vi "3 Mirror Engine.vi"(0 "Unique Notifier Name":string, 11 "DAQmx AO Lines":string[](array[string])) -> ()   [LabVIEW 2020]
uses:
  3 Mirror Scan Type Defs/3 Mirror Scan Note Type.ctl
  3 Mirror Scan Type Defs/3 Mirror Scan Actions.ctl
  3 Mirror Scan Type Defs/3 Mirror Scan Cal Data.ctl
  <vilib>/DAQmx/write.llb/DAQmx Write (Analog 1D Wfm NChan NSamp).vi
  <vilib>/DAQmx/write.llb/DAQmx Write (Analog 1D DBL NChan 1Samp).vi
  <vilib>/DAQmx/create/channels.llb/DAQmx Create Channel (AO-Voltage-Basic).vi
  <vilib>/DAQmx/configure/timing.llb/DAQmx Timing (Sample Clock).vi
  <vilib>/DAQmx/miscellaneous.llb/DAQmx Fill In Error Info.vi
  <resource>/objmgr/daqmx.rc
panel:
  out "Last Error":errorcluster
  in  "Quit":bool
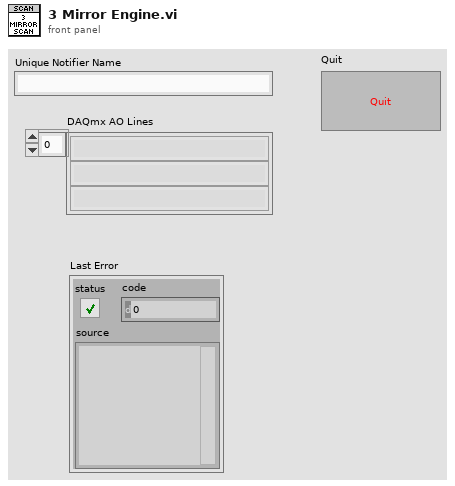
[diagram p1: front panel]
types:
  T1 = typedef "3 Mirror Scan Cal Data.ctl" = cluster{"XCenter":dbl, "YCenter":dbl, "M1_Px_Per_Volt":dbl, "M2_Px_Per_Volt":dbl, "MirrorCoupling":dbl, "Phase01":dbl, "Phase02":dbl, "Phase03":dbl}
  T2 = typedef "3 Mirror Scan Actions.ctl" = enum16{"Idle", "Scan Timed", "Scan Live", "Convert ROI", "Run Scan", "Exit Loop", "Quit"}
  T3 = typedef "3 Mirror Scan Note Type.ctl" = cluster{"Actions":T2, "Global Rectangle":i32[], "Running":bool, "Scan Frequency (Hz)":dbl, "Scan Time (s)":dbl}
  T4 = typedef "3 Mirror Scan ROI Voltage Data.ctl" = cluster{"X Freq (Hz)":dbl, "Y Freq (Hz)":dbl, "X Offset (V)":dbl, "X Amp (V)":dbl, "Y Offset (V)":dbl, "Y Amp (V)":dbl}
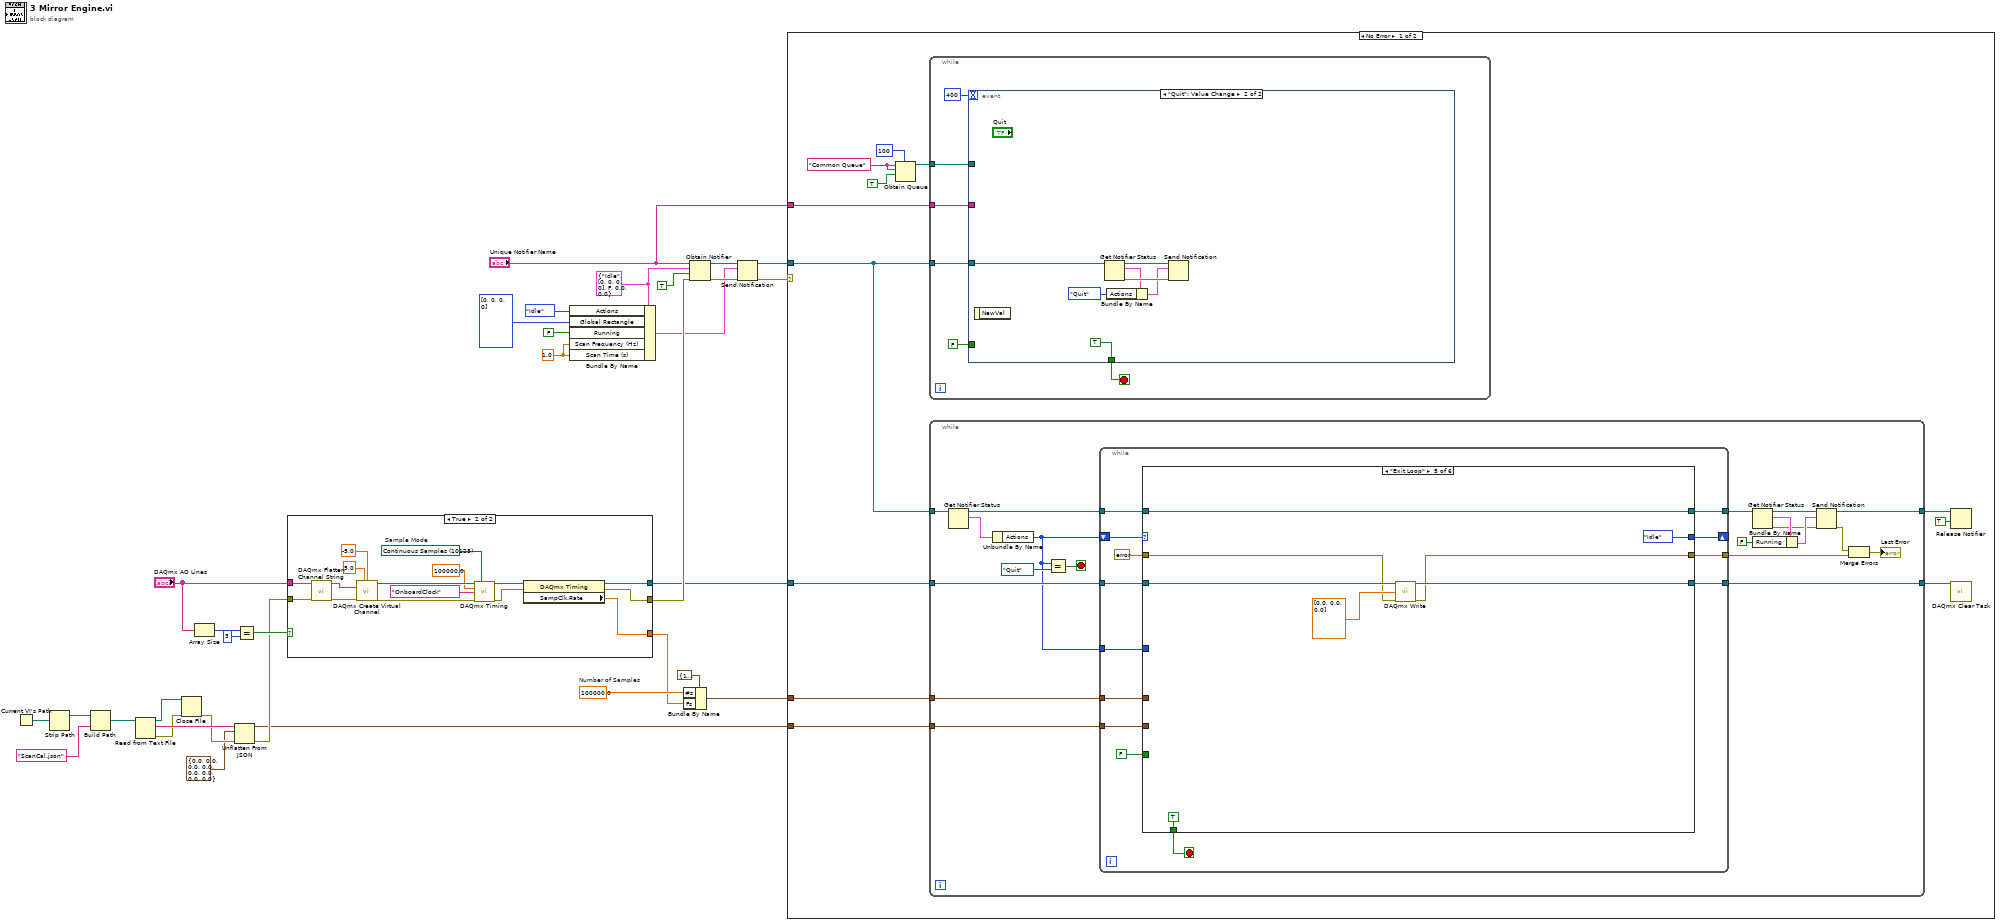
[diagram p0: block diagram]
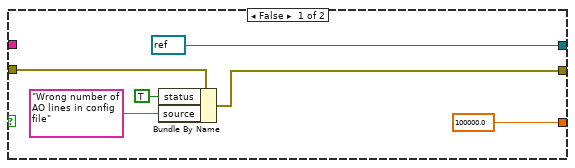
[diagram p2: hidden frame]
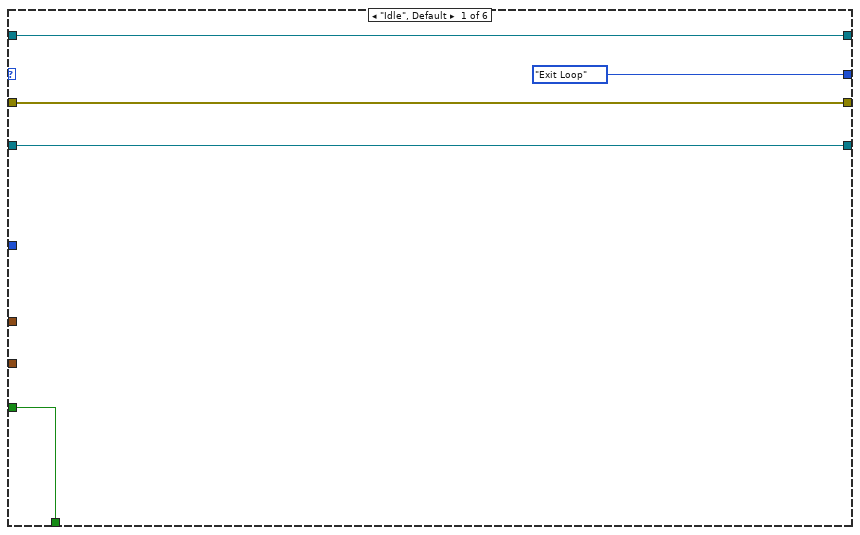
[diagram p3: hidden frame]
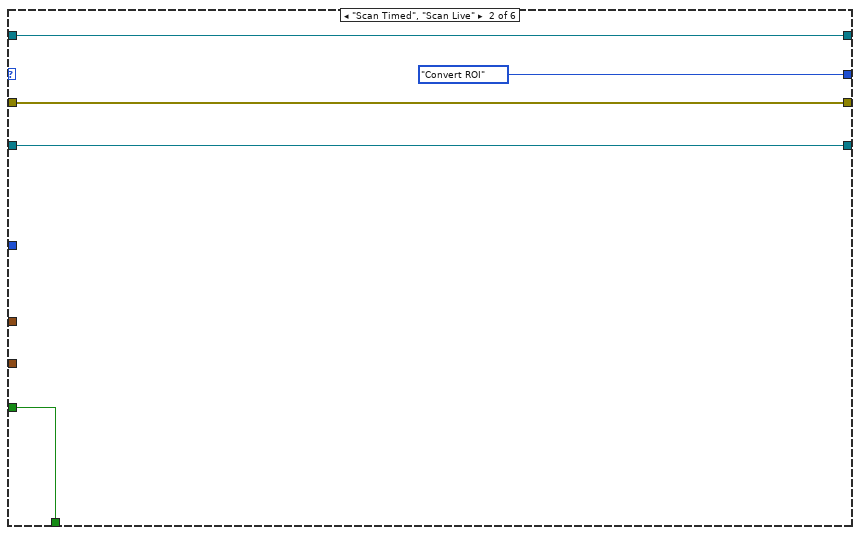
[diagram p4: hidden frame]
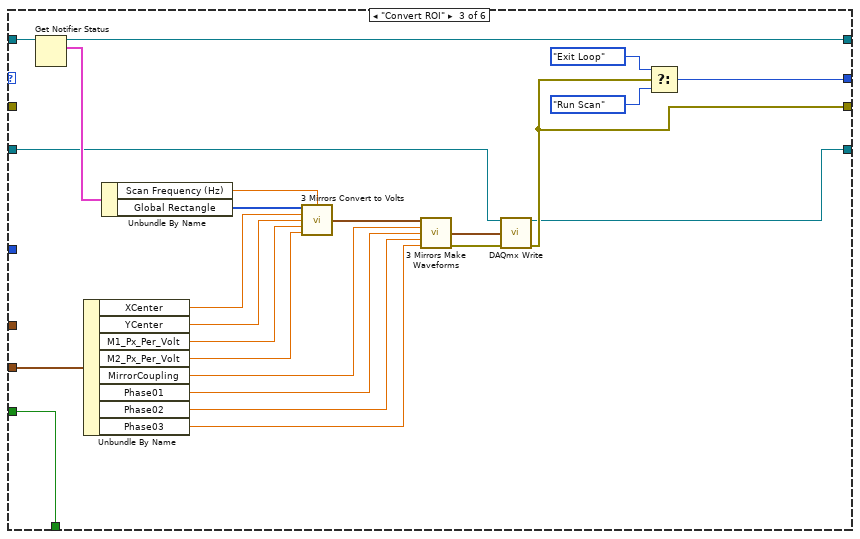
[diagram p5: hidden frame]
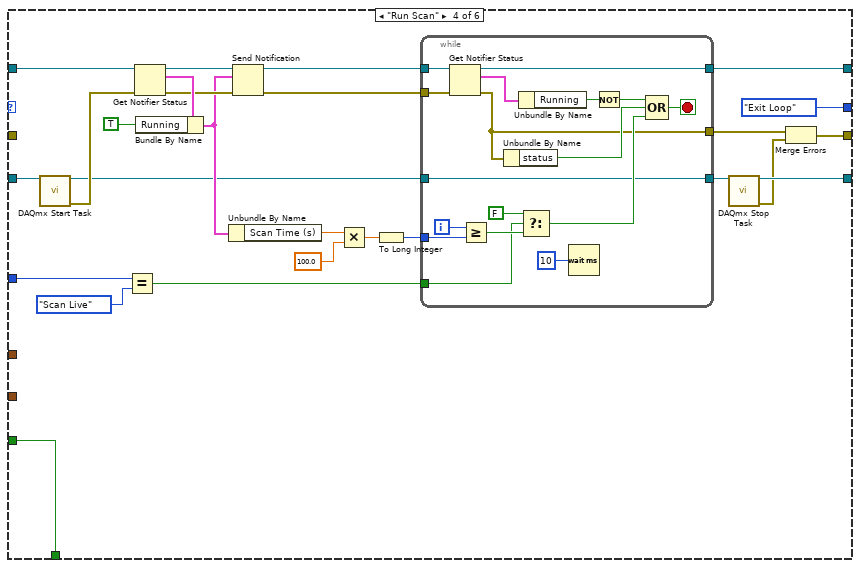
[diagram p6: hidden frame]
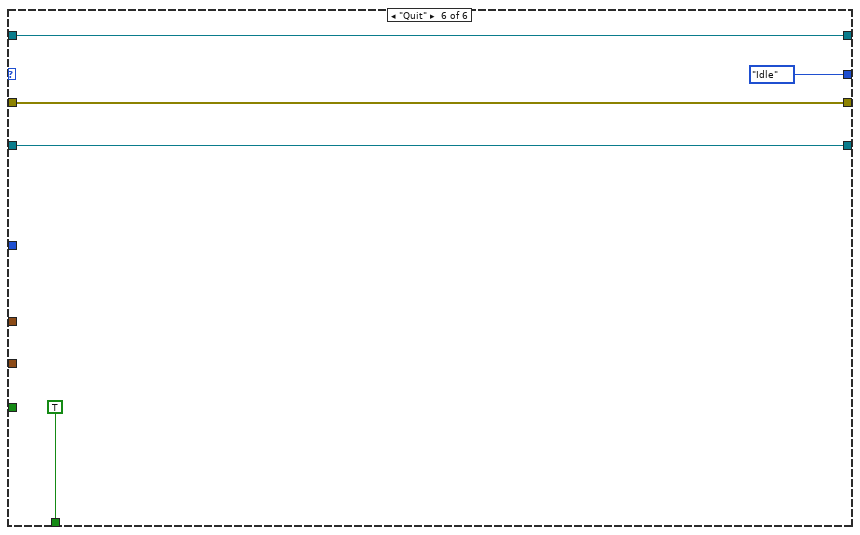
[diagram p7: hidden frame]
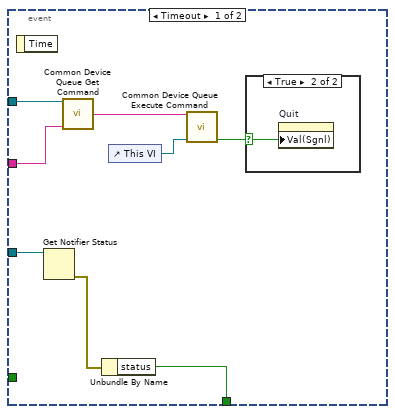
[diagram p8: hidden frame]
diagram:
  w15 = 1.0 ("Scan Frequency (Hz)")
  w19 = T3 {"Actions"=enum."Idle", "Global Rectangle"=[0, 0, 0, 0], "Running"=FALSE, "Scan Frequency (Hz)"=0.0, "Scan Time (s)"=0.0} ("3 Mirror Notifier")
  w21 = 100000.0  # Number of Samples
  n1 = Current VI's Path() -> (path=w12:path)
  n2 = Strip Path(path=w12) -> (stripped path=w11:path)  [unwired: 1 out]
  n3 = Build Path(base path=w11, name or relative path="ScanCal.json") -> (appended path=w9:path)
  n4 = Read from Text File(file (use dialog)=w9) -> (refnum out=w7:refnum<file>, text=w8:string, error out=w6:errorcluster)  [unwired: 3 in, 1 out]
  n5 = Close File(refnum=w7, error in=w6) -> (error out=w5:errorcluster)  [unwired: 1 out]
  n6 = Array Size(array="DAQmx AO Lines") -> (size(s)=w27:i32)
  n7 = Unflatten From JSON(JSON string=w8, type and defaults=T1 {"XCenter"=0.0, "YCenter"=0.0, "M1_Px_Per_Volt"=0.0, "M2_Px_Per_Volt"=0.0, "MirrorCoupling"=0.0, "Phase01"=0.0, "Phase02"=0.0, "Phase03"=0.0} ("ScanCalibration"), error in (no error)=w5) -> (value=w2:T1, error out=w3:errorcluster)  [unwired: 4 in]
  n8 = Equal?(x=w27, y=3) -> (x = y?=w25:bool)
  n9 = case shown="True" w25 {
    tunnel: "DAQmx AO Lines" -> [_ w55]
    tunnel: w3 -> [w39 w54]
    tunnel: [w35 w41] -> w23
    tunnel: [refnum<k21> refnum ("task out") w42] -> w13
    tunnel: [100000.0 ("Sample Rate") w40] -> w20
    frame False {
      n10 = Bundle By Name(cluster=w39, "status"=TRUE, "source"="Wrong number of AO lines in config file") -> (w35:errorcluster)
    }
    frame True {
      w51 = 10123 items=["Finite Samples"=10178, "Continuous Samples"=10123, "Hardware Timed Single Point"=12522]  # Sample Mode
      n11 = call <vilib>:"DAQmx Flatten Channel String.vi"("names in"=w55, "error in"=w54) -> ("names out"=w46:string, "error out"=w45:errorcluster)  [unwired: 12 in]
      n12 = call-poly <vilib>:"DAQmx Create Virtual Channel.vi"("maximum value"=5.0 ("Max Voltage"), "minimum value"=-5.0 ("Min Voltage"), "physical channels"=w46, "error in"=w45) -> ("task out"=w53:refnum<k21>, "error out"=w52:errorcluster)  [unwired: 10 in]
      n13 = call-poly <vilib>:"DAQmx Timing.vi"("task/channels in"=w53, "sample mode"=w51, "rate"=100000.0 ("Sample Rate"), "source"=tag "OnboardClock" ("Sample Clock Source"), "error in"=w52) -> ("task out"=w44:refnum<k21>, "error out"=w43:errorcluster)  [unwired: 9 in]
      n14 = property class="DAQmx Timing"(reference=w44, error in=w43) -> (reference out=w42:refnum<k21>, error out=w41:errorcluster, "SampClk.Rate"=w40:dbl)
    }
  }
  n15 = Bundle By Name(cluster=w19, "Actions"=3_Mirror_Scan_Actions."Idle", "Global Rectangle"=i32[] [0, 0, 0, 0], "Running"=FALSE, "Scan Frequency (Hz)"=w15, "Scan Time (s)"=w15) -> (w14:T3)
  n16 = Bundle By Name(cluster=cluster{"Fs":dbl, "#s":dbl} {"Fs"=1000.0, "#s"=1000.0} ("sampling info"), "#s"=w21, "Fs"=w20) -> (w1:cluster{"Fs":dbl, "#s":dbl})
  n17 = Obtain Notifier(name (unnamed)="Unique Notifier Name", notification data type=w19, create if not found? (T)=TRUE, error in (no error)=w23) -> (notifier out=w32:refnum<notifier>, error out=w31:errorcluster)  [unwired: 1 out]
  n18 = Send Notification(notification=w14, notifier=w32, error in (no error)=w31) -> (notifier out=w29:refnum<notifier>, error out=w30:errorcluster)
  n19 = case shown="No Error" w30 {
    tunnel: w29 -> [w62 _]
    tunnel: "Unique Notifier Name" -> [w63 _]
    tunnel: w13 -> [w61 _]
    tunnel: w2 -> [w58 _]
    tunnel: w1 -> [w57 _]
    frame No Error {
      w67 = "Common Queue" ("Unique Notifier Name")
      n20 = Obtain Queue(max queue size (-1, unlimited)=100, name (unnamed)=w67, element data type=w67, create if not found? (T)=TRUE) -> (queue out=w64:refnum<queue>)  [unwired: 1 in, 2 out]
      n21 = while {
        tunnel: w62 -> [w196]
        tunnel: w64 -> [w193]
        tunnel: w63 -> [w192]
        stop <- w194 stop-if-true
        n22 = event shown="[1] \"Quit\": Value Change" {
          selector: _ -> [_ _]
          dyn-events: _ -> [_ _]
          timeout: 400 -> [_ _]
          tunnel: w196 -> [w204 w207]
          tunnel: [w202 TRUE ("status")] -> w194
          tunnel: w193 -> [w198 _]
          tunnel: w192 -> [w197 _]
          tunnel: FALSE ("status") -> [_ _]
          event Timeout {
            n23 = event-data() -> ()  [unwired: 1 in, 1 out]
            n24 = Get Notifier Status(notifier=w204) -> (error out=w203:errorcluster)  [unwired: 1 in, 4 out]
            n25 = call "Common Device Queue Get Command.vi"("Common Queue"=w198, "Notifier Name"=w197) -> ("Command"=w200:string)  [unwired: 12 in, 1 out]
            n26 = Unbundle By Name(w203) -> ("status"=w202:bool)
            n27 = control-ref of="This VI"() -> (w199:refnum<vi>)
            n28 = call "Common Device Queue Execute Command.vi"("Common Command"=w200, "VI Refnum"=w199) -> ("Quit?"=w201:bool)  [unwired: 12 in, 1 out]
            n29 = case shown="True" w201 {
              selector: w201 -> [_ w205]
              frame False {
              }
              frame True {
                n30 = property on="Quit" class="Bool (strict)"("Val(Sgnl)"=w205) -> ()  [unwired: 2 in, 2 out]
              }
            }
          }
          event "Quit": Value Change {
            n31 = event-data() -> ()  [unwired: 1 in, 1 out]
            n32 = Get Notifier Status(notifier=w207) -> (notifier out=w208:refnum<notifier>, current notification=w209:T3, error out=w211:errorcluster)  [unwired: 1 in, 2 out]
            n33 = Bundle By Name(cluster=w209, "Actions"=3_Mirror_Scan_Actions."Quit") -> (w210:T3)
            n34 = Send Notification(notification=w210, notifier=w208, error in (no error)=w211) -> ()  [unwired: 2 out]
          }
        }
      }
      n35 = while {
        tunnel: w62 -> [w87]
        tunnel: w61 -> [w82]
        tunnel: [w75] -> w59
        tunnel: w58 -> [w73]
        tunnel: w57 -> [w74]
        tunnel: [w71] -> w56
        stop <- w84 stop-if-true
        n36 = Get Notifier Status(notifier=w87) -> (notifier out=w83:refnum<notifier>, current notification=w86:T3)  [unwired: 1 in, 3 out]
        n37 = Unbundle By Name(w86) -> ("Actions"=w72:T2)
        n38 = Equal?(x=w72, y=3_Mirror_Scan_Actions."Quit") -> (x = y?=w84:bool)
        n39 = while {
          shift-right: [w95] -> _
          shift-left: w72 -> [w99]
          tunnel: w83 -> [w97]
          tunnel: w82 -> [w96]
          tunnel: [w94] -> w81
          tunnel: w74 -> [w93]
          tunnel: w73 -> [w92]
          tunnel: w72 -> [w91]
          tunnel: [w90] -> w71
          tunnel: [w89] -> w70
          stop <- w98 stop-if-true
          n40 = case shown="\"Exit Loop\"" w99 {
            tunnel: FALSE -> [w105 w110 w134 w160 _ _]
            tunnel: [w105 w110 w134 w160 TRUE TRUE] -> w98
            tunnel: w97 -> [w103 w108 w133 w154 w179 w188]
            tunnel: w96 -> [w101 w106 w118 w159 w184 w187]
            tunnel: [3_Mirror_Scan_Actions."Exit Loop" ("y") 3_Mirror_Scan_Actions."Convert ROI" ("y") w114 3_Mirror_Scan_Actions."Exit Loop" ("y") 3_Mirror_Scan_Actions."Idle" ("y") 3_Mirror_Scan_Actions."Idle" ("y")] -> w95
            tunnel: [w103 w108 w131 w139 w179 w188] -> w94
            tunnel: w93 -> [_ _ _ _ _ _]
            tunnel: w92 -> [_ _ w130 _ _ _]
            tunnel: w91 -> [_ _ _ w152 _ _]
            tunnel: [w101 w106 w111 w140 w182 w187] -> w90
            tunnel: [w102 w107 w112 w135 w180 w186] -> w89
            tunnel: errorcluster {"status"=FALSE, "code"=0, "source"=""} ("error IO") -> [w102 w107 _ _ w181 w186]
            frame "Idle", Default {
            }
            frame "Scan Timed", "Scan Live" {
            }
            frame "Convert ROI" {
              n41 = Get Notifier Status(notifier=w133) -> (notifier out=w131:refnum<notifier>, current notification=w132:T3)  [unwired: 1 in, 3 out]
              n42 = Unbundle By Name(w130) -> ("XCenter"=w124:dbl, "YCenter"=w127:dbl, "M1_Px_Per_Volt"=w126:dbl, "M2_Px_Per_Volt"=w125:dbl, "MirrorCoupling"=w122:dbl, "Phase01"=w121:dbl, "Phase02"=w120:dbl, "Phase03"=w119:dbl)
              n43 = Unbundle By Name(w132) -> ("Scan Frequency (Hz)"=w128:dbl, "Global Rectangle"=w129:i32[])
              n44 = call "3 Mirrors Convert to Volts.vi"("Global Rectangle"=w129, "Scan Freq (Hz)"=w128, "X Center"=w124, "Y Center"=w127, "M1 Volts Per Px"=w126, "M2 Volts Per Px"=w125) -> ("Voltage Data"=w123:T4)  [unwired: 9 in]
              n45 = call "3 Mirrors Make Waveforms.vi"("Axis Voltage Data"=w123, "Mirror Coupling"=w122, "Phase 01"=w121, "Phase 02"=w120, "Phase 03"=w119) -> ("Waveform Data"=w117:waveform(dbl)[], "Error Out"=w116:errorcluster)  [unwired: 9 in]
              n46 = call-poly <vilib>:"DAQmx Write.vi"("task/channels in"=w118, "data"=w117, "error in"=w116) -> ("task out"=w111:refnum<k21>, "error out"=w112:errorcluster)  [unwired: 10 in, 1 out]
              n47 = Select(t=3_Mirror_Scan_Actions."Exit Loop" ("y"), s=w112, f=3_Mirror_Scan_Actions."Run Scan") -> (s? t:f=w114:T2)
            }
            frame "Run Scan" {
              n48 = call <vilib>:"DAQmx Start Task.vi"("task/channels in"=w159) -> ("task out"=w142:refnum<k21>, "error out"=w153:errorcluster)  [unwired: 13 in]
              n49 = Equal?(x=w152, y=3_Mirror_Scan_Actions."Scan Live") -> (x = y?=w146:bool)
              n50 = Get Notifier Status(notifier=w154, error in (no error)=w153) -> (notifier out=w158:refnum<notifier>, current notification=w157:T3, error out=w155:errorcluster)  [unwired: 2 out]
              n51 = Bundle By Name(cluster=w157, "Running"=TRUE) -> (w150:T3)
              n52 = Unbundle By Name(w150) -> ("Scan Time (s)"=w149:dbl)
              n53 = Send Notification(notification=w150, notifier=w158, error in (no error)=w155) -> (notifier out=w147:refnum<notifier>, error out=w143:errorcluster)
              n54 = Multiply(x=w149, y=100.0) -> (x*y=w145:dbl)
              n55 = To Long Integer(number=w145) -> (32bit integer=w144:i32)
              n56 = while {
                tunnel: w147 -> [w177]
                tunnel: w146 -> [w169]
                tunnel: [w173] -> w139
                tunnel: w144 -> [w172]
                tunnel: w143 -> [w163]
                tunnel: w142 -> [w162]
                tunnel: [w162] -> w141
                tunnel: [w161] -> w137
                i -> [w171]
                stop <- w164 stop-if-true
                n57 = Get Notifier Status(notifier=w177, error in (no error)=w163) -> (notifier out=w173:refnum<notifier>, current notification=w176:T3, error out=w161:errorcluster)  [unwired: 2 out]
                n58 = Greater Or Equal?(x=w171, y=w172) -> (x >= y?=w170:bool)
                n59 = Unbundle By Name(w161) -> ("status"=w166:bool)
                n60 = Unbundle By Name(w176) -> ("Running"=w175:bool)
                n61 = Select(t=FALSE, s=w169, f=w170) -> (s? t:f=w165:bool)
                n62 = Wait (ms)(milliseconds to wait=u32 10) -> ()  [unwired: 1 out]
                n63 = Not(x=w175) -> (.not. x?=w167:bool)
                n64 = Compound Arithmetic op=OR(w167, w166, w165) -> (w164:bool)
              }
              n65 = call <vilib>:"DAQmx Stop Task.vi"("task/channels in"=w141) -> ("task out"=w140:refnum<k21>, "error out"=w136:errorcluster)  [unwired: 13 in]
              n66 = Merge Errors(w137, w136) -> (w135:errorcluster)
            }
            frame "Exit Loop" {
              n67 = call-poly <vilib>:"DAQmx Write.vi"("task/channels in"=w184, "data"=dbl[] [0.0, 0.0, 0.0], "error in"=w181) -> ("task out"=w182:refnum<k21>, "error out"=w180:errorcluster)  [unwired: 10 in, 1 out]
            }
            frame "Quit" {
            }
          }
        }
        n68 = Get Notifier Status(notifier=w81) -> (notifier out=w80:refnum<notifier>, current notification=w79:T3, error out=w76:errorcluster)  [unwired: 1 in, 2 out]
        n69 = Bundle By Name(cluster=w79, "Running"=FALSE) -> (w77:T3)
        n70 = Send Notification(notification=w77, notifier=w80, error in (no error)=w76) -> (notifier out=w75:refnum<notifier>, error out=w69:errorcluster)
        n71 = Merge Errors(w69, w70) -> (→"Last Error":errorcluster)
      }
      n72 = Release Notifier(notifier=w59, force destroy? (F)=TRUE) -> ()  [unwired: 1 in, 3 out]
      n73 = call <vilib>:"DAQmx Clear Task.vi"("task in"=w56) -> ()  [unwired: 14 in, 1 out]
    }
    frame Error {
    }
  }
